vi "Launch LabActor.vi"() -> ()   [LabVIEW 2024]
uses:
  LabActor/LabActor.lvclass
  C:/GitHub/LabActor/Controllers/Application Controller/Application Controller.lvclass
  Controllers/Application Controller/Load App.vi
  Controllers/Application Controller/Application Controller.lvclass
panel:
  out "Build version":string
  out "Last modified":string
  out "Path":string
  out "Waiting Lights":T1
  out "Current action:":string
  # "LabActor Framework"
  # "© 2012-2026\n\nFedor F. Balakirev\nfbalakirev@gmail.com"
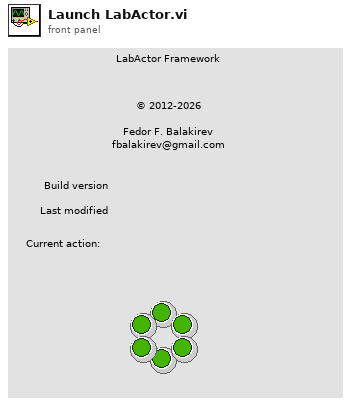
[diagram p1: front panel]
types:
  T1 = cluster{"DNL_wait 1":bool, "DNL_wait 1":bool, "DNL_wait 1":bool, "DNL_wait 1":bool, "DNL_wait 1":bool, "DNL_wait 1":bool}
  T2 = cluster{"[0]":bool, "[1]":bool, "[2]":bool, "[3]":bool, "[4]":bool, "[5]":bool}
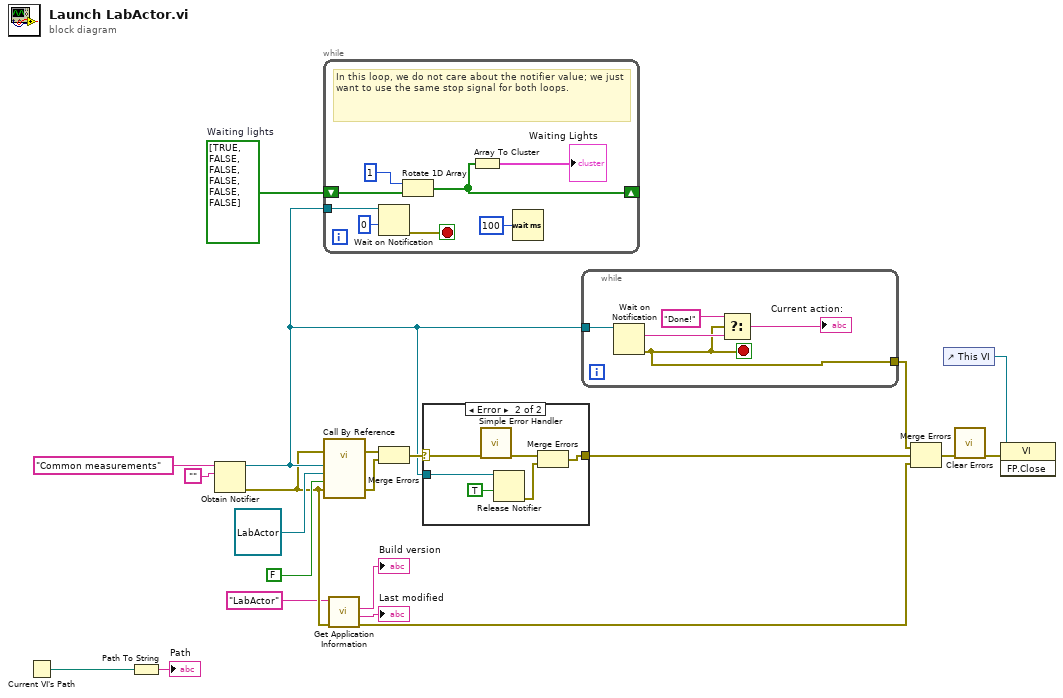
[diagram p0: block diagram]
diagram:
  w11 = bool[] [TRUE, FALSE, FALSE, FALSE, FALSE, FALSE]  # Waiting lights
  n1 = Current VI's Path() -> (path=w8:path)
  n2 = Path To String(path=w8) -> (string=→"Path":string)
  n3 = Obtain Notifier(name (unnamed)="Common measurements", notification data type="") -> (notifier out=w9:refnum<notifier>, error out=w6:errorcluster)  [unwired: 2 in, 1 out]
  n4 = while {
    shift-right: [w23] -> _
    shift-left: w11 -> [w25]
    tunnel: w9 -> [w27]
    stop <- w29 stop-if-true
    # "In this loop, we do not care about the notifier value; we just want to use the same stop signal for both loops."
    n5 = Wait on Notification(notifier=w27, timeout in ms (-1)=0) -> (error out=w29:errorcluster)  [unwired: 2 in, 3 out]
    n6 = Rotate 1D Array(1:w25, 2:1 ("n")) -> (0:w23:bool[])
    n7 = Array To Cluster(array=w23) -> (cluster=→"Waiting Lights":T2)
    n8 = Wait (ms)(milliseconds to wait=u32 100) -> ()  [unwired: 1 out]
  }
  n9 = call-by-ref "?"(error in=w6, "Error In"=w6, "Open Actor Core front panel? (F)"=FALSE, "Application Controller.lvclass"=refnum<class "LabActor.lvclass"> refnum ("LabActor.lvclass"), "Status Notifier"=w9) -> (error out=w19:errorcluster, "Error Out"=w16:errorcluster)  [unwired: 8 in, 1 out]
  n10 = call "Get Application Information.vi"("error out"=w6, "Build Name"="LabActor") -> ("Error Out"=w4:errorcluster, "Last modified"=→"Last modified":string, "Build version"=→"Build version":string)  [unwired: 5 in, 2 out]
  n11 = Merge Errors(w19, w16) -> (w20:errorcluster)
  n12 = case shown="Error" w20 {
    selector: w20 -> [w30 w36]
    tunnel: [w30 w33] -> w14
    tunnel: w9 -> [_ w35]
    frame No Error {
    }
    frame Error {
      n13 = call <vilib>:"Simple Error Handler.vi"("error in (no error)"=w36) -> ("error out"=w34:errorcluster)  [unwired: 4 in, 4 out]
      n14 = Release Notifier(notifier=w35, force destroy? (F)=TRUE) -> (error out=w32:errorcluster)  [unwired: 1 in, 2 out]
      n15 = Merge Errors(w34, w32) -> (w33:errorcluster)
    }
  }
  n16 = while {
    tunnel: w9 -> [w41]
    tunnel: [w37] -> w12
    stop <- w37 stop-if-true
    n17 = Wait on Notification(notifier=w41) -> (notification=w39:string, error out=w37:errorcluster)  [unwired: 3 in, 2 out]
    n18 = Select(t="Done!" ("notification"), s=w37, f=w39) -> (s? t:f=→"Current action:":string)
  }
  n19 = Merge Errors(w12, w14, w4) -> (w13:errorcluster)
  n20 = control-ref of="This VI"() -> (w1:refnum<vi>)
  n21 = call <vilib>:"Clear Errors.vi"("error in (no error)"=w13) -> ("error out"=w21:errorcluster)  [unwired: 5 in, 1 out]
  n22 = invoke class="VI" method="FP.Close"(reference=w1, error in=w21) -> ()  [unwired: 1 in, 3 out]
